vi "MW100_Read_GAL_Flow.vi"(0 "MW100":refnum<visa-resource-name>="MW100", 2 "Semiphore":T1, 11 "Error In":errorcluster) -> (4 "dup VISA session":refnum<visa-resource-name>, 6 "Gallons":dbl, 8 "Flow(GPM)":dbl, 10 "Tc_down":dbl, 15 "Error Out":errorcluster)   [LabVIEW 2012]
uses:
  ChannelSettings.ctl
panel:
  out "Data List":dbl[](array[numeric]) format="%.4f"
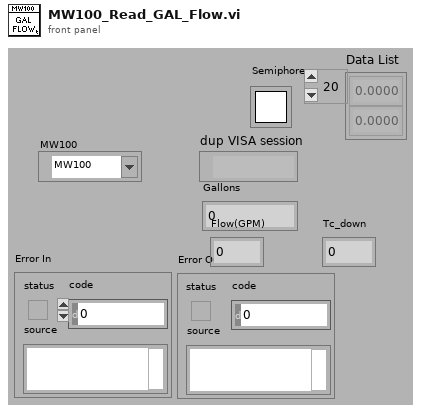
[diagram p1: front panel]
types:
  T1 = typedef "Semaphore RefNum" = refnum<k1>
  T2 = typedef "ChannelSettings.ctl" = u32
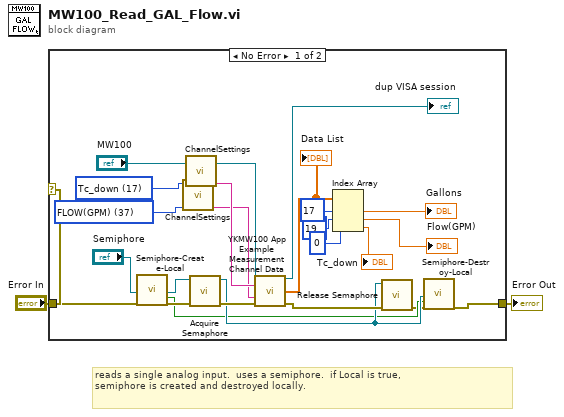
[diagram p0: block diagram]
diagram:
  # "reads a single analog input.  uses a semiphore.  if Local is true, \nsemiphore is created and destroyed locally."
  n1 = case shown="No Error" "Error In" {
    tunnel: "Error In" -> [w15 w26]
    tunnel: [w9 w26] -> w2
    frame No Error {
      w6 = T2 37 items=["4-20_OUT", "Pres_HI1", "Pres_HI2", "Pres_LOW", "Pres_PIN", "HEATER_TOP", "HEATER_BOT", "T_Shell", "FLOWMETER", "WATT_SENSE", "WH_TICK", "Tc_1", "Tc_2", "Tc_3", "Tc_4", "Tc_5", "Tc_6", "Tc_down", "T_Shell_2", "T_Shell_3", "T_Shell_4", "RTD_IN", "RTD_OUT", "RTD_AMB", "INTF_TEMPFLO", "INTF_READY", "INTF_START", "INTF_STOP", "DRM_LOW", "DRM_HIGH", "PWR_MAIN", "VLV_DUMP", "VLV_OUT", "VLV_IN", "WATT_HOURS", "FLOW(SAMPLE)", "GALLONS", "FLOW(GPM)", "FLOW_CALC_GAIN", "FLOW_CALC_OFFSET", "FLOW_CALC_THRESHOLD", "VLV_DUMP_2", "VLV_OUT_2", "VLV_IN_2", "VLV_DUMP_3", "VLV_OUT_3", "VLV_IN_3", "VLV_DUMP_4", "VLV_OUT_4", "VLV_IN_4", "CHAN_34", "CHAN_35", "CHAN_36"] ("Channel_Enum")
      w20 = T2 17 items=["4-20_OUT", "Pres_HI1", "Pres_HI2", "Pres_LOW", "Pres_PIN", "HEATER_TOP", "HEATER_BOT", "T_Shell", "FLOWMETER", "WATT_SENSE", "WH_TICK", "Tc_1", "Tc_2", "Tc_3", "Tc_4", "Tc_5", "Tc_6", "Tc_down", "T_Shell_2", "T_Shell_3", "T_Shell_4", "RTD_IN", "RTD_OUT", "RTD_AMB", "INTF_TEMPFLO", "INTF_READY", "INTF_START", "INTF_STOP", "DRM_LOW", "DRM_HIGH", "PWR_MAIN", "VLV_DUMP", "VLV_OUT", "VLV_IN", "WATT_HOURS", "FLOW(SAMPLE)", "GALLONS", "FLOW(GPM)", "FLOW_CALC_GAIN", "FLOW_CALC_OFFSET", "FLOW_CALC_THRESHOLD", "VLV_DUMP_2", "VLV_OUT_2", "VLV_IN_2", "VLV_DUMP_3", "VLV_OUT_3", "VLV_IN_3", "VLV_DUMP_4", "VLV_OUT_4", "VLV_IN_4", "CHAN_34", "CHAN_35", "CHAN_36"] ("Channel_Enum")
      n2 = call "Semiphore-Create-Local.vi"("Semiphore"="Semiphore", "error in (no error)"=w15) -> ("semaphore"=w14:T1, "Local?"=w11:bool, "error out"=w13:errorcluster)  [unwired: 15 in]
      n3 = call "ChannelSettings.vi"("Channel_Enum"=w6) -> ("Channel String"=w5:string)  [unwired: 10 in]
      n4 = call "ChannelSettings.vi"("Channel_Enum"=w20) -> ("Channel String"=w25:string)  [unwired: 10 in]
      n5 = call <vilib>:"Acquire Semaphore.vi"("error in (no error)"=w13, "semaphore"=w14) -> ("error out"=w19:errorcluster, "semaphore out"=w12:T1)  [unwired: 3 in, 1 out]
      n6 = call "YKMW100 App Example Measurement Channel Data.vi"("VISA session"="MW100", "Start Channel (001)"=w25, "End Channel (001)"=w5, "error in (no error)"=w19) -> ("dup VISA session"=→"dup VISA session":refnum<visa-resource-name>, "Data List"=w22:dbl[], "error out"=w18:errorcluster)  [unwired: 4 in, 5 out]
      "Data List" <- w22
      n7 = Index Array(array=w22, index #1=17 ("index"), index #2=19 ("index"), index #3=0 ("index")) -> (element #1=→"Gallons":dbl, element #2=→"Flow(GPM)":dbl, element #3=→"Tc_down":dbl)
      n8 = call <vilib>:"Release Semaphore.vi"("error in (no error)"=w18, "semaphore"=w12) -> ("error out"=w10:errorcluster)  [unwired: 4 in, 1 out]
      n9 = call "Semiphore-Destroy-Local.vi"("Semiphore"=w12, "Local?"=w11, "error in (no error)"=w10) -> ("error out"=w9:errorcluster)  [unwired: 16 in]
    }
    frame Error {
    }
  }
  "Error Out" <- w2
